vi "SetParam.vi"(8 "error in (no error)":errorcluster caption="entrée d'erreur (pas d'erreur)", 10 "fetch_20newsgroups_vectorized":T1={"subset"="train", "remove"=[], "download_if_missing"=TRUE, "normalize"=TRUE, "Returns"="Data"}, 11 "20newsgroups_vectorized.lvclass":refnum<class "20newsgroups_vectorized.lvclass">) -> (0 "error out":errorcluster caption="sortie d'erreur", 3 "20newsgroups_vectorized.lvclass":refnum<class "20newsgroups_vectorized.lvclass">)   [LabVIEW 2020, in "20newsgroups_vectorized.lvclass"]
doc: "Set Parameters"
uses:
  20newsgroups_vectorized.lvclass
  20newsgroups_vectorized.lvclass/20newsgroups_vectorized.ctl
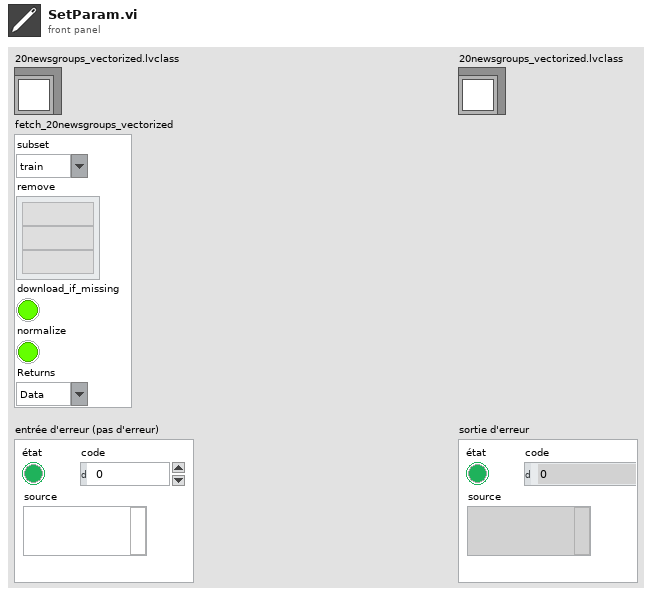
[diagram p1: front panel]
types:
  T1 = cluster{"subset":string, "remove":string[], "download_if_missing":bool, "normalize":bool, "Returns":string}
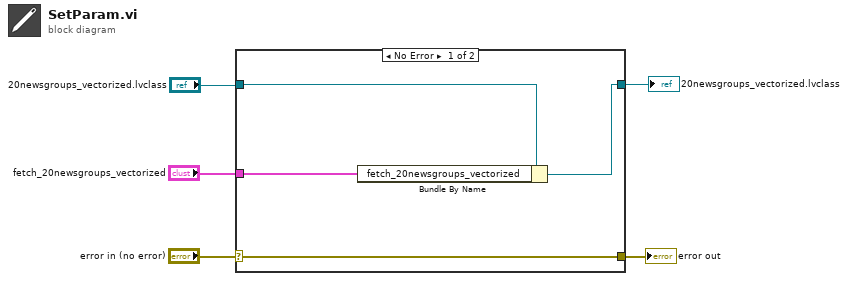
[diagram p0: block diagram]
diagram:
  n1 = case shown="No Error" "error in (no error)" {
    selector: "error in (no error)" -> [w9 w10]
    tunnel: [w9 w10] -> w4
    tunnel: [w7 w11] -> w1
    tunnel: "20newsgroups_vectorized.lvclass" -> [w8 w11]
    tunnel: "fetch_20newsgroups_vectorized" -> [w6 _]
    frame No Error {
      n2 = Bundle By Name(cluster=w8, "fetch_20newsgroups_vectorized"=w6) -> (w7:refnum<class "20newsgroups_vectorized.lvclass">)
    }
    frame Error {
    }
  }
  "error out" <- w4
  "20newsgroups_vectorized.lvclass" <- w1
